vi "PTScanner.parse data descriptor.vi"(0 "dataDescriptor":T1) -> (14 "Input Parameters":T2(array[cluster]), 16 "Output Parameters":T2(array[cluster]), 19 "Comment":string)   [LabVIEW 2014, in "PTScanner.lvlib"]
uses:
  PTScanner.lvlib
  CSCore/BaseProcess/BaseProcess.descriptor string definition.ctl
  CSCore/CSSystem/CoreLib/CoreLib.lvlib
  CSCore/BaseProcess/BaseProcess.lvlib
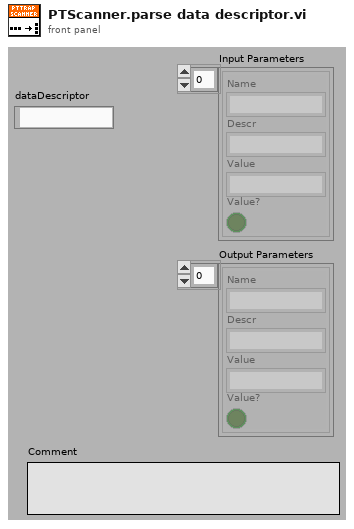
[diagram p1: front panel]
types:
  T1 = typedef "BaseProcess.lvlib/BaseProcess.descriptor string definition.ctl" = string
  T2 = cluster{"Name":string, "Descr":string, "Value":string, "Value?":bool}[]
  T3 = cluster{"Data Descriptor":string, "inputDescriptor":string, string, bool}
  T4 = cluster{"Data Descriptor":string, "inputDescriptor":string, "Value":string, "Value?":bool}[]
  T5 = cluster{"Data Descriptor":string, "inputDescriptor":string, "Value":string, "Value?":bool}
  T6 = cluster{"Data Descriptor":string, "outputDescriptor":string, string, bool}
  T7 = cluster{"Data Descriptor":string, "outputDescriptor":string, "Value":string, "Value?":bool}[]
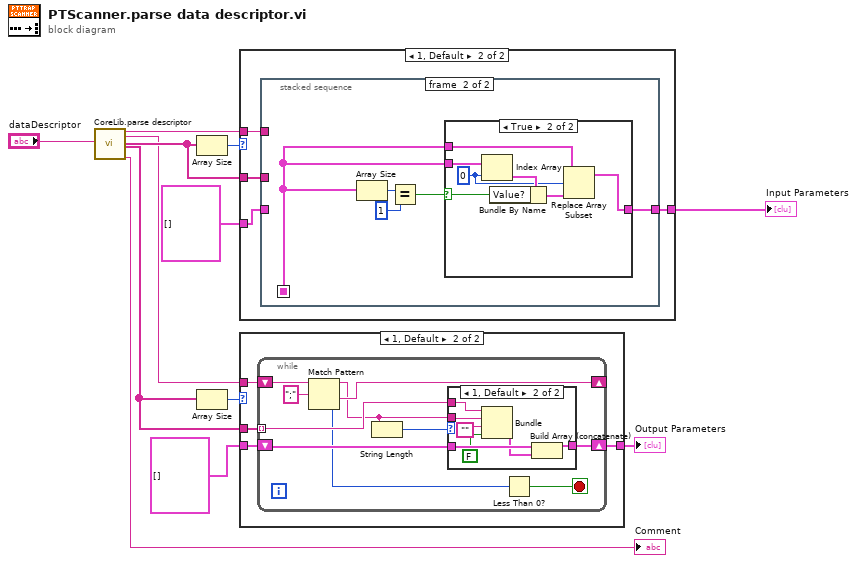
[diagram p0: block diagram]
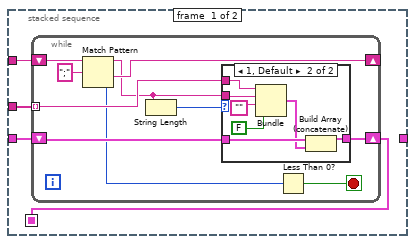
[diagram p5: hidden frame]
diagram:
  n1 = call "CoreLib.parse descriptor.vi"("dataDescriptor"="dataDescriptor") -> ("inputDescriptor"=w12:string, "outputDescriptor"=w6:string, "inputNames"=w10:string[], "outputNames"=w4:string[], "comment"=→"Comment":string)  [unwired: 13 in, 1 out]
  n2 = Array Size(array=w10) -> (size(s)=w9:i32)
  n3 = Array Size(array=w4) -> (size(s)=w7:i32)
  n4 = case shown="1, Default" w9 {
    tunnel: w12 -> [_ w16]
    tunnel: [_ w13] -> w8
    tunnel: w10 -> [_ w15]
    tunnel: T2 [] ("Input Parameter 2") -> [_ w14]
    frame 0 {
    }
    frame 1, Default {
      n5 = stacked-sequence {
        seq-local: [w17 _] -> [_ w40]
        tunnel: w16 -> [w20 _]
        tunnel: w15 -> [w19 _]
        tunnel: w14 -> [w18 _]
        tunnel: [_ w39] -> w13
        frame #0 {
          n6 = while {
            tunnel: w19 -> [w29] mode=indexing
            shift-right: [w25] -> _
            shift-left: w20 -> [w30]
            shift-right: [w28] -> w17
            shift-left: w18 -> [w27]
            stop <- w24 stop-if-true
            n7 = Match Pattern(string=w30, regular expression=";") -> (before substring=w22:string, after substring=w25:string, offset past match=w23:i32)  [unwired: 1 in, 1 out]
            n8 = String Length(string=w22) -> (length=w21:i32)
            n9 = case shown="1, Default" w21 {
              tunnel: w29 -> [_ w38]
              tunnel: [w31 w36] -> w28
              tunnel: w27 -> [w31 w35]
              tunnel: w22 -> [_ w37]
              frame 0 {
              }
              frame 1, Default {
                n10 = Bundle("Data Descriptor"=w38, "inputDescriptor"=w37, "", FALSE) -> (w34:T3)  [unwired: 1 in]
                n11 = Build Array (concatenate)(w35, w34) -> (w36:T4)
              }
            }
            n12 = Less Than 0?(x=w23) -> (x < 0?=w24:bool)
          }
        }
        frame #1 {
          n13 = Array Size(array=w40) -> (size(s)=w43:i32)
          n14 = Equal?(x=w43, y=1) -> (x = y?=w41:bool)
          n15 = case shown="True" w41 {
            selector: w41 -> [_ w50]
            tunnel: w40 -> [w44 w48]
            tunnel: w40 -> [_ w47]
            tunnel: [w44 w45] -> w39
            frame False {
            }
            frame True {
              w46 = 0
              n16 = Index Array(array=w48, index=w46) -> (element=w51:T5)
              n17 = Bundle By Name(cluster=w51, "Value?"=w50) -> (w49:T5)
              n18 = Replace Array Subset(array=w47, new element=w49, index=w46) -> (w45:T4)
            }
          }
        }
      }
    }
  }
  "Input Parameters" <- w8
  n19 = case shown="1, Default" w7 {
    tunnel: w6 -> [_ w55]
    tunnel: [_ w54] -> w5
    tunnel: w4 -> [_ w53]
    tunnel: T2 [] ("Input Parameter 2") -> [_ w52]
    frame 0 {
    }
    frame 1, Default {
      n20 = while {
        tunnel: w53 -> [w64] mode=indexing
        shift-right: [w60] -> _
        shift-left: w55 -> [w65]
        shift-right: [w63] -> w54
        shift-left: w52 -> [w62]
        stop <- w59 stop-if-true
        n21 = Match Pattern(string=w65, regular expression=";") -> (before substring=w57:string, after substring=w60:string, offset past match=w58:i32)  [unwired: 1 in, 1 out]
        n22 = String Length(string=w57) -> (length=w56:i32)
        n23 = case shown="1, Default" w56 {
          tunnel: w64 -> [_ w73]
          tunnel: [w66 w71] -> w63
          tunnel: w62 -> [w66 w70]
          tunnel: w57 -> [_ w72]
          frame 0 {
          }
          frame 1, Default {
            n24 = Bundle("Data Descriptor"=w73, "outputDescriptor"=w72, "", FALSE) -> (w69:T6)  [unwired: 1 in]
            n25 = Build Array (concatenate)(w70, w69) -> (w71:T7)
          }
        }
        n26 = Less Than 0?(x=w58) -> (x < 0?=w59:bool)
      }
    }
  }
  "Output Parameters" <- w5
